vi "Refresh with loaded ROI.vi"(7 "ROI fit info cluster":T1 {"ROI fit info"."Frame size"."Old" items=["100X100"=100, "128X128"=128, "200X200"=200, "256X256"=256, "512X512"=512, "1024x1024"=1024, "2048x2048"=2048]; "ROI fit info"."Frame size"."New" items=["100X100"=100, "128X128"=128, "200X200"=200, "256X256"=256, "512X512"=512, "1024x1024"=1024, "2048x2048"=2048]}, 10 "Old ROI file's data":dbl[][](array[numeric]), 11 "Old ROI file path":path) -> (1 "Last ROI Enum":T3, 3 "Proceed?":bool)   [LabVIEW 2017]
uses:
  Typedefs/ROI ID Enum.ctl
  Typedefs/ROI fitting info cluster.ctl
  Typedefs/Frame Size.ctl
  Typedefs/ROI management FG states.ctl
panel:
  out "No ROI":bool
  out "Number of ROI":i32
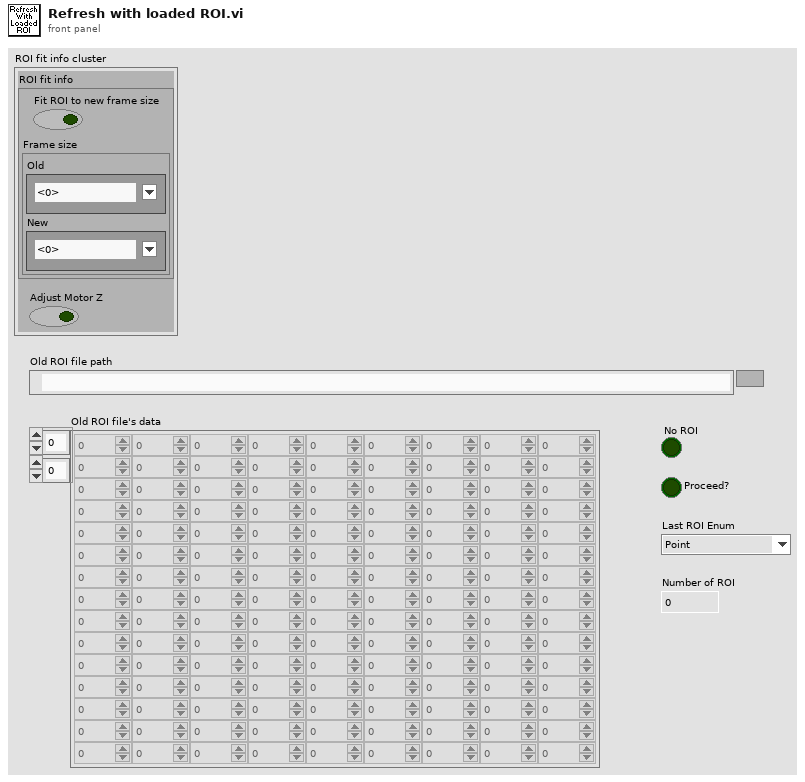
[diagram p1: front panel]
types:
  T1 = typedef "ROI fitting info cluster.ctl" = cluster{"ROI fit info":cluster{"Fit ROI to new frame size":bool, "Frame size":cluster{"Old":T2, "New":T2}}, "Adjust Motor Z":bool}
  T2 = typedef "Frame Size.ctl" = u16
  T3 = typedef "ROI ID Enum.ctl" = enum16{"Point", "MiniScan", "Comp. MiniScan", "Rectangle", "Comp. volume", "Arb. plane point"}
  T4 = typedef "ROI management FG states.ctl" = enum16{"Read", "Write", "Write-from dataset", "Clear Last", "Clear All", "Update ROIs time", "Reload last ROI set", "Offset all ROI", "Offset visible ROI"}
  T5 = typedef "ROI spec.ctl" = cluster{"Coordinates":i32[], "Zoom":dbl, "ROI Enum":T3, "Z planeIdx(s)":i32[], "Z planecodes(s)":u8[], "Z start":dbl, "Z stop":dbl}
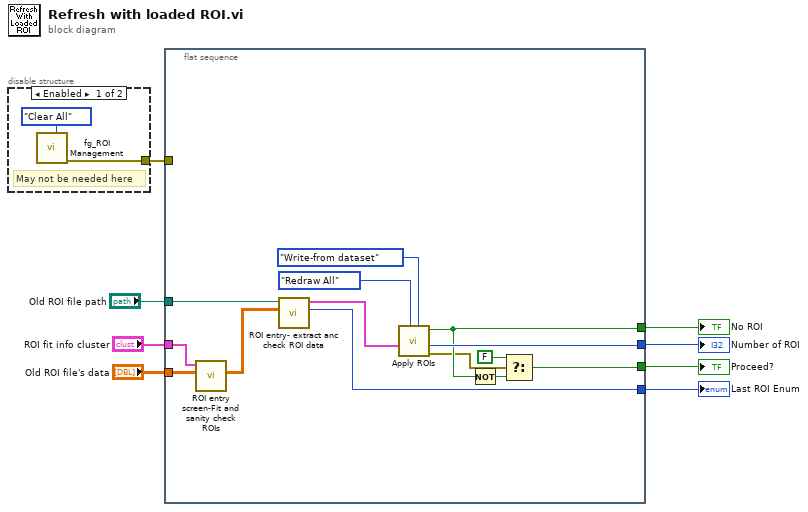
[diagram p0: block diagram]
diagram:
  n1 = disable-structure shown="Enabled" {
    disable-tunnel: [w9 _] -> w1
    frame Enabled {
      # "May not be needed here"
      n2 = call "fg_ROI Management.vi"("Function"=ROI_management_FG_states."Clear All") -> ("error out"=w9:errorcluster)  [unwired: 6 in, 4 out]
    }
    frame Disabled {
    }
  }
  n3 = flat-sequence {
    tunnel: "Old ROI file path" -> [w15]
    tunnel: [w24] -> w7
    tunnel: [w12] -> w6
    tunnel: [w23] -> w5
    tunnel: [w22] -> w4
    tunnel: "Old ROI file's data" -> [w21]
    tunnel: "ROI fit info cluster" -> [w20]
    tunnel: w1 -> [_]
    frame #0 {
      n4 = call "ROI entry screen-Fit and sanity check ROIs.vi"("Old ROI file's data in"=w21, "ROI fit info"=w20) -> ("Fitted ROI data"=w14:dbl[][])  [unwired: 9 in]
      n5 = call "ROI entry- extract anc check ROI data.vi"("ROI File data"=w14, "Old ROI file path"=w15) -> ("Last ROI Enum"=w12:T3, "Array"=w13:T5[])  [unwired: 5 in, 3 out]
      n6 = call "Apply ROIs.vi"("Function"=ROI_management_FG_states."Write-from dataset", "Mode (Redraw All)"=enum16{"Redraw All", "Draw Last"}."Redraw All", "ROIs Info []"=w13) -> ("error out"=w18:errorcluster, "Number of ROI"=w23:i32, "No ROI"=w22:bool)  [unwired: 5 in, 1 out]
      n7 = Not(x=w22) -> (.not. x?=w17:bool)
      n8 = Select(t=FALSE, s=w18, f=w17) -> (s? t:f=w24:bool)
    }
  }
  "Proceed?" <- w7
  "Last ROI Enum" <- w6
  "Number of ROI" <- w5
  "No ROI" <- w4
